vi "AlliGator Compute Phasor Plot Weber 2-Component Decomposition.vi"(5 "Lifetime Graph refnum":refnum<vi>, 8 "error in (no error)":errorcluster, 11 "AlliGator IV DVR":refnum<data-value>) -> (0 "error out":errorcluster, 1 "Message":string, 3 "AlliGator IV DVR":refnum<data-value>)   [LabVIEW 2021, in "AlliGator Phasor Plot.lvlib"]
doc: "Computes the 2-component linear decomposition of each phasor using Weber's apparoach.\n\nReturns two scatter plots (tau 2 vs tau 1 and f1 vs tau 1) sent to the Lifetime Graph."
uses:
  AlliGator Phasor Plot.lvlib
  Internal Variables/AlliGator Internal Variables v2.ctl
  <vilib>/vision/Image Controls.llb/IMAQ Image.ctl
  Internal Variables/AlliGator Gate Image Set.ctl
  Files/AlliGator FLI Dataset Type.ctl
  Files/AlliGator Data Series Type.ctl
  Dual-Channel Datasets/AlliGator Dataset Channel.ctl
  Settings/AlliGator Gate Arithmetic.ctl
  Source Image/AlliGator Displayed Image.ctl
  Image/Named ROI Description.ctl
  Phasor Graph/AlliGator Decay Metadata v3.ctl
  Decay Analysis/Decay Preprocessing/AlliGator Decay Background Subtraction Info.ctl
  Decay Analysis/Decay Preprocessing/AlliGator Baseline Subtraction Method.ctl
  Graphs/XY Graph/XY Graph Plot Shift Parameters.ctl
  Graphs/XY Graph/XY Graph Plot Shift Method.ctl
  Decay Analysis/Decay Preprocessing/AlliGator Decay Extrapolation Parameters.ctl
  Phasor/Calibration Phasor (m, phi).ctl
  Phasor/Phasor Reference Series.ctl
  Phasor/Phasor Calibration Map v2.ctl
  Phasor/Phasor (g, s).ctl
  Phasor Graph/AlliGator Raw Phasor Plot Data v4.ctl
  Phasor/Phasor Standard Deviation Options.ctl
  AlliGator Phasor Multi-Harmonic Data.ctl
  Phasor/Phasor Harmonic Data.ctl
  Decay Fit Parameter Map/AlliGator Decay Fit Options & Parameters v2.ctl
  Fits/IRF(X)PSED/Decay Fit Options v2.ctl
  Fits/Decay Convolution/Decay Model.ctl
  Fits/Residual Type.ctl
  Fits/IRF(X)PSED/Fit Weights Type.ctl
  Fits/Non-linear Fitting Method v2.ctl
  Fits/Fit Calculation Method.ctl
  Fits/Non-linear Fitting Algorithm.ctl
  Decay Analysis/Decay Fit/AlliGator Decay Fit Parameter Constraints 2.ctl
  Fits/IRF(X)PSED/Decay Fit Parameters In List.ctl
  Fits/IRF(X)PSED/MLE Baseline Offset Type.ctl
  Decay Analysis/Decay Preprocessing/AlliGator Decay Preprocessing Parameters.ctl
  Fits/IRF(X)PSED/Decay Fit Parameters & Derived Quantities List v2.ctl
  Decay Fit Parameter Map/AlliGator Parameter Maps Data.ctl
  Globals, Variables, Constants/AlliGator Variables List.ctl
  Variant/Variant to Data/Variant to [I32].vi
  Graphs/XY Graph/XY Graph Add-Ons.lvlib
  Phasor/Phasor.lvlib
  Error/Error.lvlib
  Globals, Variables, Constants/AlliGator Globals, Variables & Constants.lvlib
  Variant/Variant to Data/Variant to Data.lvlib
  Phasor Harmonic/AlliGator Phasor Harmonics.lvlib
  Image/Image.lvlib
  Decay Analysis/Decay Preprocessing/AlliGator Decay Preprocessing.lvlib
  Phasor Graph/AlliGator Phasor Graph.lvlib
  Files/AlliGator Files.lvlib
  Internal Variables/AlliGator Internal Variables.lvlib
  Source Image/AlliGator Source Image.lvlib
  Fits/Fits.lvlib
  Decay Analysis/Decay Fit/AlliGator Decay Fit.lvlib
  Decay Fit Parameter Map/AlliGator Decay Fit Parameter Map.lvlib
  Settings/AlliGator Settings.lvlib
  Dual-Channel Datasets/AlliGator Dual-Channel Datasets.lvlib
panel:
  # "see the AlliGator License on the block diagram (Ctrl+E or Window:Show Block Diagram)"
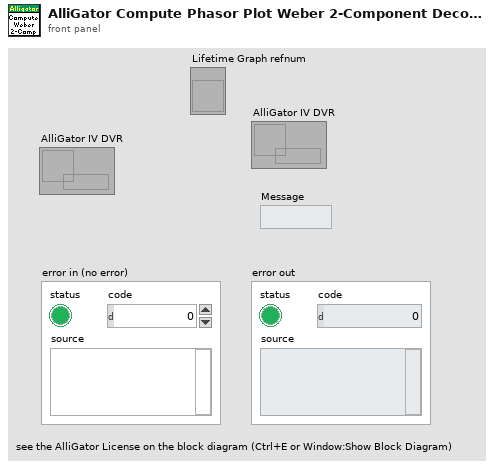
[diagram p1: front panel]
types:
  T1 = typedef "Phasor.lvlib/Phasor Harmonic Data.ctl" = cluster{"Phasor Harmonic Name":string, "Phasor Plot Settings Checksum":u64, "Phasor Frequency":dbl[unit], "Base Frequency":dbl[unit], "Harmonic Order":u8, "Phasor Plot Parameters":string, "Phasor Array [[CSG]]":csg[][], "Dataset File Path":path}
  T2 = typedef "AlliGator Globals, Variables & Constants.lvlib/AlliGator Variables List.ctl" = enum16{"---- GUI ----", "GUI:Initialization Status", "GUI:State Indicators Refnum", "GUI:Original AlliGator Menu Items", "GUI:Current Action Loop State", "GUI:Script in progress", "GUI:Playback", "GUI:Loop Playback", "GUI:Search ROI Used", "GUI:Search ROI", "Decay Graph Max Legend Size", "Intensity Graph Max Legend Size", "Decay Statistics Graph Max Legend Size", "Phasor Graph Max Legend Size", "Phasor Ratio Graph Max Legend Size", "Lifetime Graph Max Legend Size", "---- Files ----", "Files:Export Dataset Frames as Individual Files", "Files:Show Batch Export Help Balloons", "Files:Frames in Dataset", "Files:ptu File Frame Start Indices", "Files:Current Frame in Dataset", "Files:Current Frame Timestamp", "Files:Dataset Loaded", "Files:Dataset Metadata", "Files:Dataset Channel", "Files:Dataset Data Description", "Files:Background Dataset Metadata", "Files:Background Dataset Channel", "Files:Background Dataset Data Description", "Files:Background File Subtraction", "Files:Background File Path", "Files:Background File Pile-up Correction", "Files:Background File Pixel Well Capacity", "Files:Background File Scaling Factor", "Files:Current Dataset Load Settings", "Files:Dataset Path", "Files:ICCD-specific Information", "Files:Macrotime Gate Separation", "------ Python Plugins ------", "Python Plugins:Information", "Python Plugins:Python Session", "Python Plugins:Valid Python Session?", "---- Source Image ----", "Source Image:ROIs", "Source Image:Current ROI", "Source Image:ROI Event Refnum", "X_Source Image:Display Range", "X_Source Image:Palette Information", "X_Source Image:Type of Displayed Image", "X_Time Gate Slider", "Source Image:Palette List", "Source Image:Scale", "Source Image:ROI Overlay Color", "Source Image:Overlay to Erase", "Source Image:Is Displayed Image Accumulated", "Source Image:White Light Image Modified", "Source Image:Mask Image Modified", "---- Image Profile Window ----", "Image Profile:Window Event Refnum", "Image Profile:IntensityType", "Image Profile:Intensity Average Type", "Image Profile:Intensity-weighted SDV", "Image Profile:Box Profile Type", "Image Profile:Window Open", "Image Profile:Plotted Fit Parameter", "------ Phasor Graph -------", "Phasor Graph:Show Line", "---- Phasor Plot ---", "Phasor Plot:Parameters Changed", "Phasor Plot:FLI Dataset Modified since last Calculation", "Phasor Harmonics Data", "Selected Phasor Harmonics", "Phasor Harmonic Manager Event Refnum", "Phasor Plot:ROIs", "Phasor Plot:Current ROI", "Phasor Plot:ROI Event Refnum", "Phasor Plot:Image Reference Points", "Phasor Plot:Computed", "Phasor Plot:Palette Information", "Phasor Plot:Palette List", "Phasor Plot:Phasor Ratio Palette Information", "Phasor Plot:Phasor Ratio Palette List", "Phasor Plot:Image Scale", "Phasor Plot:Image Overlay to Erase", "Phasor Plot:Image Elements to Update", "Phasor Plot:Current Calculation Parameters", "Phasor Plot:Current Calibration Options", "Phasor Plot:Reset Cumulated Phasor Plot", "Phasor Plot:Reference 1", "Phasor Plot:Lifetime Reference 1", "Phasor Plot:Reference 1 Frequency", "Phasor Plot:Reference 2", "Phasor Plot:Lifetime Reference 2", "Phasor Plot:Reference 2 Frequency", "---- Decay Analysis ----", "Number of Selected Decays to Fit", "LS Fit Results", "LAR Fit Results", "BS Fit Results", "Last Decay Max - Min", "Best Fit Parameters", "Best Fit Parameter Names", "Actual Size X", "Actual Size Y", "Binning X", "Binning Y", "Actual # Gates", "Dataset Number", "Gates to...", "Gates Skipped", "Gates to keep", "Gate Step", "Gate Separation", "Reversed Gates", "Pile-up Correction", "Pixel Well Capacity", "Background Subtracted", "Background Subtraction Method", "Background Definition Range", "Background File (deprecated)", "Number of Dataset Accumulated", "Array of Accumulated Dataset Paths", "Do Averaged Datasets", "Destination File Path", "Process Plot Target", "Use 1/D as Phasor Frequency", "---- Decay Fit Parameter Map -----", "Decay Fit Parameter Map:Palette Information", "Decay Fit Parameter Map:Palette List", "Decay Fit Parameter Map:X Resolution", "Decay Fit Parameter Map:Y Resolution", "---- Parameter Map ----", "Parameter Map:Palette Information", "Parameter Map:Palette List", "------- Local Decay Window ---------", "Local Decay Graph Window:Event Refnum", "Local Decay Graph Window:Use normalized IRF for convolution", "----- Miscellaneous ----", "Misc:Skippable Dialog Windows Status"}
  T3 = typedef "AlliGator Internal Variables.lvlib/AlliGator Internal Variables v2.ctl" = cluster{"Displayed Image":T4, "White Light Image":T4, "Mask Image":T4, "ROI Mask Image":T4, "Current Dataset Images 1":T5, "Background Dataset Images 1":T5, "Current Dataset Images 2":T5, "Background Dataset Images 2":T5, "Current Dataset Arithmetic Images":T5, "Accumulated Dataset Images 1":T5, "Accumulated Dataset Images 2":T5, "Accumulated Dataset Arithmetic Images":T5, "Phasor Plot Image":T4, "Decay Fit Parameter Map Image":T4, "Parameter Map Image":T4, "Single Data Point Path":path, "White Light Image Path":path, "Mask Image Path":path, "Time-Series Folder":path, "[Time-Series Paths]":path[], "Current Dataset":i32, "Single Dataset Type":T6, "Current Folder":string, "AlliGator Data Series Type":T7, "# Datasets":i32, "Dual-Channel Dataset":bool, "Selected Channel Name":string, "Dataset Channel":T8, "Channel Arithmetic":T9, "Dual-Channel Background Dataset":bool, "Background Channel":T8, "Dual-Channel Accumulated Dataset":bool, "Start Time":dbl, "[Time-Series Timestamps]":dbl[], "[Intensity Corrections]":dbl[], "Time Series Script":bool, "Type of Displayed Image":T10, "Gate Image Slide":u16, "# Gates":i32, "ROIs":T11[], "ROI Decay":cluster{"t Array":dbl[], "I Array":dbl[]}, "Valid Decay":bool, "Decay  Metadata":T13, "Reference Decay Plot Name":string, "Reference Decay":cluster{"t Array":dbl[], "I Array":dbl[]}, "Decay Shift Plot":cluster{"Time Stamps":dbl[], "Decay Shifts":dbl[]}, "[Decays Max Values]":sgl[], "[Decays Min Values]":sgl[], "Calibration Phasor":T19, "Calibration Phasor Series":T20, "Phasor Calibration Map":T21, "Calibration Map MD5 Digest":string, "Last Raw Phasor":T22, "Last Calibrated Phasor":T22, "Last Calibrated Phasor SDV":T22, "Phasor Graph:Phasor Plot":cluster{"g Array":dbl[], "s Array":dbl[]}, "Phasor Graph:Phasor SDV Plot":cluster{"g Array":dbl[], "s Array":dbl[]}, "[Phasor Graph:Raw Phasor Plots]":T23[], "Phasor Plot locked to Ref 1":i32, "[Phasor Plot(s) locked to Ref 1]":i32[], "[Phasor Plot(s) locked to Ref 2]":i32[], "[Pixel Phasors]":T22[], "[[Sum Image]]":dbl[][], "[[CSG Phasors]]":csg[][], "[[Valid Pixel?]]":bool[][], "I/m/phi Dataset":cluster{"I/m/phi Dataset?":bool, "Base Frequency":dbl[unit], "Harmonic Orders":u8[]}, "Multi Phasor Plot Data":T25, "Decay Fit Options & Parameters":T26, "Fit Options: Decay Preprocessing Parameters":T37, "Fit Options: Reference Decay":cluster{"t Array":dbl[], "I Array":dbl[]}, "Is Full Image Parameters Map":bool, "Is Single-Pixels Parameters Map":bool, "NLSF Parameters Map X Resolution":i32, "NLSF Parameters Map Y Resolution":i32, "[Single Decay Fit Parameters]":dbl[], "Fit Model":T28, "[[Multiple Decays Fit Parameters]]":dbl[][], "[[Multiple Decays Fit Parameter SDVs]]":dbl[][], "[[IRFs]]":dbl[][], "IRF Array Time Axis":dbl[], "Decay Array Time Axis":dbl[], "[Decay Fit Parameter Names]":T38[], "[[Phasor Ratios]]":dbl[][], "[[Average Lifetimes]]":dbl[][], "Amplitude Weighted Average Lifetime":bool, "[Decay Sum]":dbl[], "[Map Set Names]":string[], "[Parameter Maps]":T39[], "[[User-defined Quantities]]":dbl[][], "User-defined Quantity":string}
  T4 = typedef "IMAQ Image.ctl" = refnum<image>
  T5 = typedef "AlliGator Internal Variables.lvlib/AlliGator Gate Image Set.ctl" = cluster{"SGL Image Max":T4, "SGL Image Sum":T4, "SGL Gate Images":T4[], "SGL Image Min":T4}
  T6 = typedef "AlliGator Files.lvlib/AlliGator FLI Dataset Type.ctl" = enum16{"HDF5 FLI Dataset", "Gate Image Folder", ".sdt FLI Dataset (Becker & Hickl)", ".ptu FLI Dataset (PicoQuant)", "SS1 FLI Dataset", "SS2 FLI Dataset", "I/m/phi Dataset", ".bin FLI Dataset (PicoQuant Binned)", ".bin FLI Dataset (Piccolo Binned)", ".mat FLI Dataset"}
  T7 = typedef "AlliGator Files.lvlib/AlliGator Data Series Type.ctl" = enum16{"Not a Supported Series", "Gate Images Folder Series", "SwissSPAD 2 Dataset Series", "B&H FLI Dataset Series", "PicoQuant PTU FLI Dataset Series", "PicoQuant BIN FLI Dataset Series", "Piccolo hist BIN FLI Dataset Series", "HDF5 FLI Dataset Series"}
  T8 = typedef "AlliGator Dual-Channel Datasets.lvlib/AlliGator Dataset Channel.ctl" = enum16{"G2", "INT"}
  T9 = typedef "AlliGator Settings.lvlib/AlliGator Gate Arithmetic.ctl" = enum16{"None", "INT-G2", "G2/INT*<INT>", "(1 - G2/INT)*<INT>"}
  T10 = typedef "AlliGator Source Image.lvlib/AlliGator Displayed Image.ctl" = enum16{"Single Gate", "Sum of All Gates", "Max of All Gates", "Min of All Gates", "-", "White Ligth Image", "Mask Image"}
  T11 = typedef "Image.lvlib/Named ROI Description.ctl" = cluster{"ROI Descriptor":T12, "ROI Name":string, "Overlay Color":u32}
  T12 = typedef "ROI Descriptor" = cluster{"Global Rectangle":i32[], "Contours":cluster{"ID":enum32{"External", "Internal"}, "Type":u32, "Coordinates":i32[]}[]}
  T13 = typedef "AlliGator Phasor Graph.lvlib/AlliGator Decay Metadata v3.ctl" = cluster{"ROI Descriptor":T12, "ROI Center":cluster{"X":i32, "Y":i32}, "Decay Background Subtraction Info":T14, "Decay Reverted":bool, "Decay Smoothened":bool, "Decay Straightened":bool, "Fitted Tau (Decay Straightening)":dbl, "Decay Shift Parameters":T16, "Decay Shifted":bool, "Decay Extrapolated":bool, "Decay Extrapolation Parameters":T18, "Decay Normalized":bool, "Fold Decay":bool, "# Folds":u32}
  T14 = typedef "AlliGator Decay Preprocessing.lvlib/AlliGator Decay Background Subtraction Info.ctl" = cluster{"Laser Period":dbl[unit], "Gate Duration":dbl[unit], "Baseline Subtraction Method":T15, "Background Definition Range":cluster{"Min Gate":dbl[unit], "Max Gate":dbl[unit]}, "Total Intensity w/o Bkgd Subtraction":dbl, "Bkgd-subtracted Intensity (exp)":dbl, "# Data Points":i32, "Background/Gate":dbl, "Fitted Lifetime":dbl[unit], "Bkgd-subtracted Intensity (theo)":dbl}
  T15 = typedef "AlliGator Decay Preprocessing.lvlib/AlliGator Baseline Subtraction Method.ctl" = enum16{"Mean", "Min", "Square Gated Single-Exponential", "File", "Constant"}
  T16 = typedef "XY Graph Add-Ons.lvlib/XY Graph Plot Shift Parameters.ctl" = cluster{"Type":T17, "Shift":dbl[unit], "Threshold":dbl, "Rotate":bool}
  T17 = typedef "XY Graph Add-Ons.lvlib/XY Graph Plot Shift Method.ctl" = enum16{"Default", "CFD", "Threshold", "Cross-Correlation"}
  T18 = typedef "AlliGator Decay Preprocessing.lvlib/AlliGator Decay Extrapolation Parameters.ctl" = cluster{"Additional Points":u32, "Head Fraction":dbl, "Fitted Tau":dbl, "Use Periodicity":bool, "Use Cursors":bool, "Tail Fraction":dbl}
  T19 = typedef "Phasor.lvlib/Calibration Phasor (m, phi).ctl" = cluster{"m":dbl, "phi":dbl, "Phasor Frequency":dbl[unit], "Reference Lifetime":dbl[unit]}
  T20 = typedef "Phasor.lvlib/Phasor Reference Series.ctl" = cluster{"m Array":dbl[], "phi Array":dbl[], "Phasor Frequency":dbl[unit], "Calibration Lifetime":dbl[unit]}
  T21 = typedef "Phasor.lvlib/Phasor Calibration Map v2.ctl" = cluster{"Phasor Frequency":dbl[unit], "Calibration Lifetime":dbl[unit], "ROI Centers":cluster{"X":i32, "Y":i32}[], "ROI Descriptors":T12[], "Map Resolution X":i32, "Map Resolution Y":i32, "z Array":cdb[]}
  T22 = typedef "Phasor.lvlib/Phasor (g, s).ctl" = cluster{"g":dbl, "s":dbl}
  T23 = typedef "AlliGator Phasor Graph.lvlib/AlliGator Raw Phasor Plot Data v4.ctl" = cluster{"Phasor Plot Name":string, "Raw Phasor Plot":T22[], "Phasor Frequency":dbl[unit], "[Decay Metadata]":T13[], "Raw Phasor Plot SDV":T22[], "Phasor SDV Options":T24, "[Calibration Phasor]":T19[]}
  T24 = typedef "Phasor.lvlib/Phasor Standard Deviation Options.ctl" = cluster{"Compute Estimated SDV":bool, "# Replicas":u32, "Use Estimated Average Phasor":bool}
  T25 = typedef "AlliGator Phasor Plot.lvlib/AlliGator Phasor Multi-Harmonic Data.ctl" = cluster{"Base Frequency":dbl[unit], "# Harmonics":u8, "Harmonic Orders":u8[], "Phasor Plot Settings Checksum":u64, "Phasor Harmonic Data Array":T1[]}
  T26 = typedef "AlliGator Decay Fit Parameter Map.lvlib/AlliGator Decay Fit Options & Parameters v2.ctl" = cluster{"SYNC Period":dbl[unit], "Fit Options":T27, "Fit Parameter Constraints":T34[], "MLE Baseline Offset":dbl, "MLE Baseline Offset Type":T36}
  T27 = typedef "Fits.lvlib/Decay Fit Options v2.ctl" = cluster{"Show Fit Residuals":bool, "Fit Model":T28, "Residual Type":T29, "Max Decay Percentile":dbl, "Min Decay Percentile":dbl, "Show Full Decay":bool, "Weights":T30, "Fitting Method":T31, "Compute Parameter Uncertainties":bool, "Periodic Boundaries":bool, "Model Calculation":T32, "Period":dbl[unit], "Termination Criteria":cluster{"Max Iterations":i32, "Max Function Calls":i32, "Max Time":dbl[unit], "Function Tolerance":dbl, "Parameter Tolerance":dbl, "Gradient Tolerance":dbl, "Min Lambda":dbl, "Max Lambda":dbl, "Initial Tick Count":u32}, "Offset Resolution":dbl[unit], "Use Local IRF":bool, "Fitting Algorithm":T33}
  T28 = typedef "Fits.lvlib/Decay Model.ctl" = enum16{"1-Exponential", "2-Exponentials"}
  T29 = typedef "Fits.lvlib/Residual Type.ctl" = enum16{"Standard", "Normalized", "Reduced"}
  T30 = typedef "Fits.lvlib/Fit Weights Type.ctl" = enum16{"Unweighted", "1/Variance", "Best of All"}
  T31 = typedef "Fits.lvlib/Non-linear Fitting Method v2.ctl" = enum16{"Least Square", "Least Absolute Residual", "Bisquare", "MLE", "-", "Best of All"}
  T32 = typedef "Fits.lvlib/Fit Calculation Method.ctl" = enum16{"Simulation", "Convolution", "Integration"}
  T33 = typedef "Fits.lvlib/Non-linear Fitting Algorithm.ctl" = enum16{"Levenberg-Marquardt", "Trust-Region Dogleg"}
  T34 = typedef "AlliGator Decay Fit.lvlib/AlliGator Decay Fit Parameter Constraints 2.ctl" = cluster{"Fit Parameter":T35, "Min Value":dbl, "Max Value":dbl, "Global":bool, "Used":bool}
  T35 = typedef "Fits.lvlib/Decay Fit Parameters In List.ctl" = enum16{"Offset", "Baseline", "A_1", "tau_1", "A_2", "tau_2"}
  T36 = typedef "Fits.lvlib/MLE Baseline Offset Type.ctl" = enum32{"Absolute", "Percentage"}
  T37 = typedef "AlliGator Decay Preprocessing.lvlib/AlliGator Decay Preprocessing Parameters.ctl" = cluster{"Background Subtraction":bool, "Straighten Decay":bool, "Reverse Gates":bool, "1-Normalized Decay":bool, "Smoothen Decay":bool, "Smoothing Parameter":dbl, "Shift Decay":bool, "Decay Shift Parameters":T16, "Extrapolate Decay":bool, "Additional Points":u32, "Head Fraction":dbl, "Pixel-Normalize Decay":bool, "Use Periodicity":bool, "Use Cursors":bool, "Tail Fraction":dbl, "Use Decay Pre-Processing":bool, "Fold Decay":bool, "# Folds":u32, "[0-1]-Normalized Decay":bool}
  T38 = typedef "Fits.lvlib/Decay Fit Parameters & Derived Quantities List v2.ctl" = enum16{"Offset", "Baseline", "A_1", "tau_1", "A_2", "tau_2", "<tau>_a", "f1_a", "f2_a", "<tau>_i", "f1_i", "f2_i", "-", "R^2", "Chi^2"}
  T39 = typedef "AlliGator Decay Fit Parameter Map.lvlib/AlliGator Parameter Maps Data.ctl" = cluster{"Map Set Name":string, "[Parameter Names]":string[], "[[Parameters]]":dbl[][], "[[Parameter SDVs]]":dbl[][], "Decay Array Time Axis":dbl[], "[[IRFs]]":dbl[][], "IRF Array Time Axis":dbl[]}
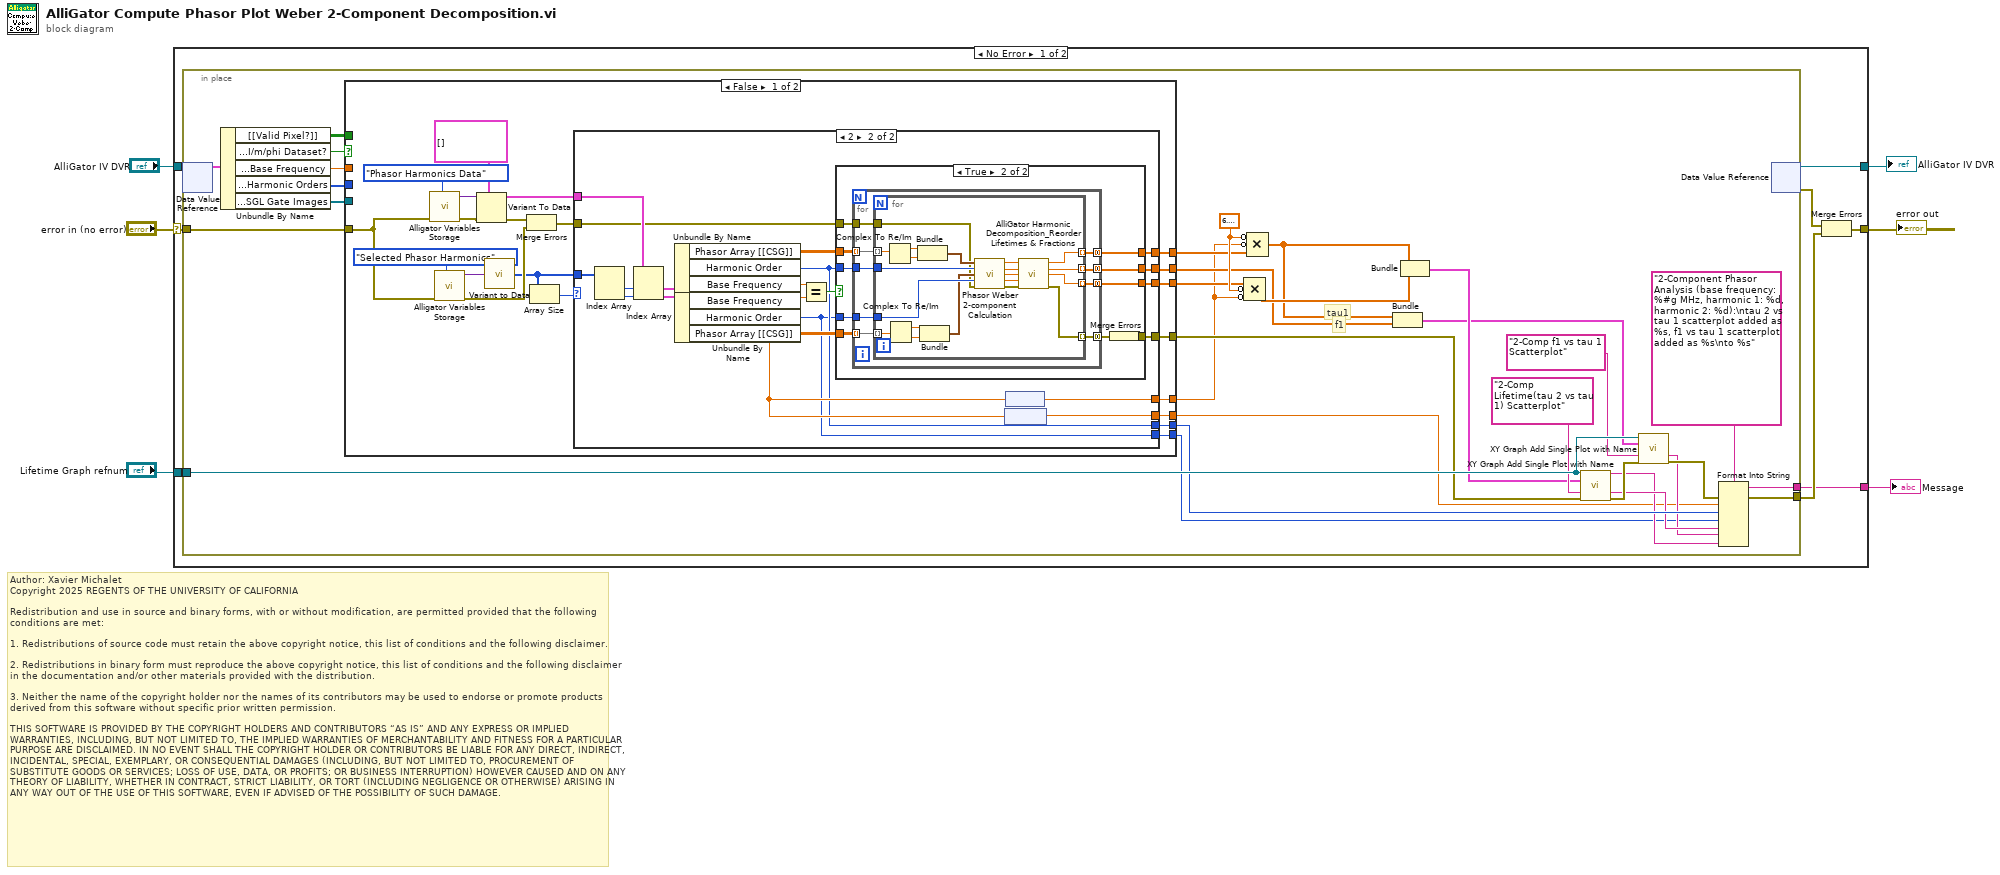
[diagram p0: block diagram]
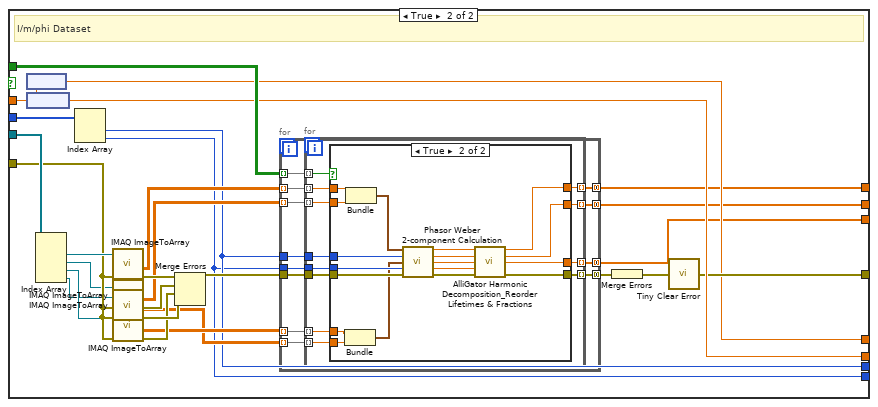
[diagram p4: hidden frame]
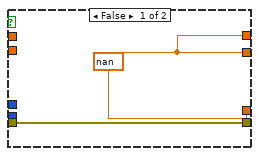
[diagram p5: hidden frame]
diagram:
  # "Author: Xavier Michalet\nCopyright 2025 REGENTS OF THE UNIVERSITY OF CALIFORNIA\n\nRedistribution and use in source and binary forms, with or without modification, are permitted provided that the following conditions are met:\n\n1. Redistributions of source code must retain the above copyright notice, this list of conditions and the following disclaimer.\n\n2. Redistributions in binary form must reproduce the above copyright notice, this list of conditions and the following disclaimer in the documentation and/or other materials provided with the distribution.\n\n3. Neither the name of the copyright holder nor the names of its contributors may be used to endorse or promote products derived from this software without specific prior written permission.\n\nTHIS SOFTWARE IS PROVIDED BY THE COPYRIGHT HOLDERS AND CONTRIBUTORS “AS IS” AND ANY EXPRESS OR IMPLIED WARRANTIES, INCLUDING, BUT NOT LIMITED TO, THE IMPLIED WARRANTIES OF MERCHANTABILITY AND FITNESS FOR A PARTICULAR PURPOSE ARE DISCLAIMED. IN NO EVENT SHALL THE COPYRIGHT HOLDER OR CONTRIBUTORS BE LIABLE FOR ANY DIRECT, INDIRECT, INCIDENTAL, SPECIAL, EXEMPLARY, OR CONSEQUENTIAL DAMAGES (INCLUDING, BUT NOT LIMITED TO, PROCUREMENT OF SUBSTITUTE GOODS OR SERVICES; LOSS OF USE, DATA, OR PROFITS; OR BUSINESS INTERRUPTION) HOWEVER CAUSED AND ON ANY THEORY OF LIABILITY, WHETHER IN CONTRACT, STRICT LIABILITY, OR TORT (INCLUDING NEGLIGENCE OR OTHERWISE) ARISING IN ANY WAY OUT OF THE USE OF THIS SOFTWARE, EVEN IF ADVISED OF THE POSSIBILITY OF SUCH DAMAGE."
  n1 = case shown="No Error" "error in (no error)" {
    selector: "error in (no error)" -> [w10 w198]
    tunnel: "AlliGator IV DVR" -> [w14 w199]
    tunnel: [w13 w199] -> w5
    tunnel: [w9 w198] -> w1
    tunnel: "Lifetime Graph refnum" -> [w11 _]
    tunnel: [w7 _] -> w2
    frame No Error {
      n2 = in-place {
        in-place-border: w11 -> [w44]
        in-place-border: w10 -> [w43]
        in-place-border: [w42] -> w8
        in-place-border: [w41] -> w7
        w24 = 6.283185307179586
        # "f1"
        # "tau1"
        n3 = in-place-dvr #1(w14) -> (w45:T3)  [unwired: 1 out]
        n4 = Unbundle By Name(w45) -> ("[[Valid Pixel?]]"=w38:bool[][], "I/m/phi Dataset.I/m/phi Dataset?"=w25:bool, "I/m/phi Dataset.Base Frequency"=w37:dbl[unit], "I/m/phi Dataset.Harmonic Orders"=w39:u8[], "Current Dataset Images 1.SGL Gate Images"=w40:T4[])
        n5 = case shown="False" w25 {
          tunnel: w40 -> [_ w153]
          tunnel: w39 -> [_ w152]
          tunnel: w38 -> [_ w151]
          tunnel: w43 -> [w61 w149]
          tunnel: w37 -> [_ w135]
          tunnel: [w48 w134] -> w16
          tunnel: [w47 w133] -> w31
          tunnel: [w50 w132] -> w27
          tunnel: [w46 w130] -> w26
          tunnel: [w53 w128] -> w21
          tunnel: [w52 w127] -> w20
          tunnel: [w51 w126] -> w19
          tunnel: [w49 w129] -> w15
          frame False {
            n6 = call "Alligator Variables Storage.vi"("AlliGator Variable"=AlliGator_Variables_List."Phasor Harmonics Data" ("Alligator Variable"), "Error In"=w61) -> ("Error Out"=w63:errorcluster, "Data out"=w62:variant)  [unwired: 7 in, 1 out]
            n7 = call "Alligator Variables Storage.vi"("AlliGator Variable"=AlliGator_Variables_List."Selected Phasor Harmonics" ("Alligator Variable"), "Error In"=w61) -> ("Error Out"=w56:errorcluster, "Data out"=w64:variant)  [unwired: 7 in, 1 out]
            n8 = Variant To Data(error in=w63, type=T1[] [] ("Array"), Variant=w62) -> (data=w58:T1[], error out=w57:errorcluster)
            n9 = call-poly "Variant to Data.vi"("Variant"=w64) -> ("Value"=w54:i32[])  [unwired: 8 in]
            n10 = Merge Errors(w57, w56) -> (w55:errorcluster)
            n11 = Array Size(array=w54) -> (size(s)=w59:i32)
            n12 = case shown="2" w59 {
              tunnel: w58 -> [_ w85]
              tunnel: w55 -> [_ w72]
              tunnel: w54 -> [_ w86]
              tunnel: [_ w76] -> w53
              tunnel: [_ w75] -> w52
              tunnel: [_ w74] -> w51
              tunnel: [_ w73] -> w50
              tunnel: [_ w71] -> w49
              tunnel: [_ w69] -> w48
              tunnel: [_ w68] -> w47
              tunnel: [_ w67] -> w46
              frame 0, Default {
              }
              frame 2 {
                n13 = Index Array(array=w86) -> (element #1=w84:i32, element #2=w83:i32)  [unwired: 2 in]
                n14 = Index Array(array=w85, index #1=w84, index #2=w83) -> (element #1=w82:T1, element #2=w81:T1)
                n15 = Unbundle By Name(w82) -> ("Phasor Array [[CSG]]"=w77:csg[][], "Harmonic Order"=w68:u8, "Base Frequency"=w80:dbl[unit])
                n16 = Unbundle By Name(w81) -> ("Base Frequency"=w70:dbl[unit], "Harmonic Order"=w67:u8, "Phasor Array [[CSG]]"=w78:csg[][])
                n17 = Equal?(x=w80, y=w70) -> (x = y?=w79:bool)
                n18 = case shown="True" w79 {
                  tunnel: w68 -> [_ w96]
                  tunnel: w67 -> [_ w95]
                  tunnel: w78 -> [_ w93]
                  tunnel: w77 -> [_ w94]
                  tunnel: [_ w92] -> w76
                  tunnel: [_ w91] -> w75
                  tunnel: [_ w90] -> w74
                  tunnel: [_ w88] -> w73
                  tunnel: w72 -> [_ w87]
                  frame False {
                  }
                  frame True {
                    n19 = for {
                      tunnel: w96 -> [w105]
                      tunnel: w95 -> [w104]
                      tunnel: w94 -> [w103] mode=indexing
                      tunnel: w93 -> [w102] mode=indexing
                      tunnel: [w101] -> w92 mode=concatenating
                      tunnel: [w100] -> w91 mode=concatenating
                      tunnel: [w99] -> w90 mode=concatenating
                      tunnel: [w98] -> w89 mode=concatenating
                      tunnel: w87 -> [w97]
                      n20 = for {
                        tunnel: w105 -> [w121]
                        tunnel: w104 -> [w120]
                        tunnel: w103 -> [w119] mode=indexing
                        tunnel: w102 -> [w118] mode=indexing
                        tunnel: [w111] -> w101 mode=indexing
                        tunnel: [w110] -> w100 mode=indexing
                        tunnel: [w109] -> w99 mode=indexing
                        tunnel: [w107] -> w98 mode=indexing
                        tunnel: w97 -> [w106]
                        n21 = Complex To Re/Im(x + iy=w119) -> (x=w117:sgl, y=w116:sgl)
                        n22 = Complex To Re/Im(x + iy=w118) -> (x=w114:sgl, y=w113:sgl)
                        n23 = Bundle(w117, w116) -> (w115:cluster{sgl, sgl})  [unwired: 1 in]
                        n24 = Bundle(w114, w113) -> (w112:cluster{sgl, sgl})  [unwired: 1 in]
                        n25 = call "Phasor Weber 2-component Calculation.vi"("Phasor 1 (g, s)"=w115, "Harmonic Order 1"=w121, "Phasor 2 (g, s)"=w112, "Harmonic Order 2"=w120, "Error In"=w106) -> ("Reduced Lifetime 1"=w125:dbl, "Fraction 1"=w123:dbl, "Reduced Lifetime 2"=w124:dbl, "Fraction 2"=w122:dbl, "Error Out"=w108:errorcluster)  [unwired: 6 in]
                        n26 = call "AlliGator Harmonic Decomposition_Reorder Lifetimes & Fractions.vi"("Reduced Lifetime 1"=w125, "Fraction 1"=w123, "Reduced Lifetime 2"=w124, "Fraction 2"=w122, "Error In"=w108) -> ("Smallest Reduced Lifetime (1)"=w111:dbl, "Fraction 1"=w110:dbl, "Largest Reduced Lifetime (2)"=w109:dbl, "Error Out"=w107:errorcluster)  [unwired: 6 in, 1 out]
                      }
                    }
                    n27 = Merge Errors(w89) -> (w88:errorcluster)
                  }
                }
                n28 = node(w70) -> (w69:dbl)
                n29 = node(w70) -> (w71:dbl)
              }
            }
          }
          frame True {
            # "I/m/phi Dataset"
            n30 = node(w135) -> (w129:dbl)
            n31 = node(w135) -> (w134:dbl)
            n32 = Index Array(array=w153) -> (element #1=w150:T4, element #2=w148:T4, element #3=w147:T4, element #4=w146:T4)  [unwired: 4 in]
            n33 = Index Array(array=w152) -> (element #1=w133:u8, element #2=w130:u8)  [unwired: 2 in]
            n34 = call "IMAQ ImageToArray"("error in (no error)"=w149, "Image"=w150) -> ("Image Pixels (Float)"=w140:sgl[][], "error out"=w145:errorcluster)  [unwired: 2 in, 3 out]
            n35 = call "IMAQ ImageToArray"("error in (no error)"=w149, "Image"=w148) -> ("Image Pixels (Float)"=w139:sgl[][], "error out"=w142:errorcluster)  [unwired: 2 in, 3 out]
            n36 = call "IMAQ ImageToArray"("error in (no error)"=w149, "Image"=w146) -> ("Image Pixels (Float)"=w137:sgl[][], "error out"=w144:errorcluster)  [unwired: 2 in, 3 out]
            n37 = call "IMAQ ImageToArray"("error in (no error)"=w149, "Image"=w147) -> ("Image Pixels (Float)"=w138:sgl[][], "error out"=w143:errorcluster)  [unwired: 2 in, 3 out]
            n38 = Merge Errors(w145, w142, w143, w144) -> (w141:errorcluster)
            n39 = for {
              tunnel: w133 -> [w165]
              tunnel: w130 -> [w164]
              tunnel: w151 -> [w163] mode=indexing
              tunnel: [w162] -> w128 mode=concatenating
              tunnel: [w161] -> w126 mode=concatenating
              tunnel: [w160] -> w127 mode=concatenating
              tunnel: w141 -> [w159]
              tunnel: w140 -> [w158] mode=indexing
              tunnel: w139 -> [w157] mode=indexing
              tunnel: w138 -> [w156] mode=indexing
              tunnel: w137 -> [w155] mode=indexing
              tunnel: [w154] -> w136 mode=concatenating
              n40 = for {
                tunnel: w165 -> [w177]
                tunnel: w164 -> [w176]
                tunnel: w163 -> [w166] mode=indexing
                tunnel: [w175] -> w162 mode=indexing
                tunnel: [w174] -> w161 mode=indexing
                tunnel: [w173] -> w160 mode=indexing
                tunnel: w159 -> [w172]
                tunnel: w158 -> [w171] mode=indexing
                tunnel: w157 -> [w170] mode=indexing
                tunnel: w156 -> [w169] mode=indexing
                tunnel: w155 -> [w168] mode=indexing
                tunnel: [w167] -> w154 mode=indexing
                n41 = case shown="True" w166 {
                  tunnel: w177 -> [_ w197]
                  tunnel: w176 -> [_ w196]
                  tunnel: [w178 w188] -> w175
                  tunnel: [w178 w186] -> w174
                  tunnel: [w178 w183] -> w173
                  tunnel: w172 -> [w179 w195]
                  tunnel: w171 -> [_ w194]
                  tunnel: w170 -> [_ w193]
                  tunnel: w169 -> [_ w191]
                  tunnel: w168 -> [_ w190]
                  tunnel: [w179 w180] -> w167
                  frame False {
                    w178 = nan ("Reduced Lifetime 1")
                  }
                  frame True {
                    n42 = Bundle(w191, w190) -> (w189:cluster{sgl, sgl})  [unwired: 1 in]
                    n43 = Bundle(w194, w193) -> (w192:cluster{sgl, sgl})  [unwired: 1 in]
                    n44 = call "Phasor Weber 2-component Calculation.vi"("Phasor 1 (g, s)"=w192, "Harmonic Order 1"=w197, "Phasor 2 (g, s)"=w189, "Harmonic Order 2"=w196, "Error In"=w195) -> ("Reduced Lifetime 1"=w187:dbl, "Fraction 1"=w184:dbl, "Reduced Lifetime 2"=w185:dbl, "Fraction 2"=w182:dbl, "Error Out"=w181:errorcluster)  [unwired: 6 in]
                    n45 = call "AlliGator Harmonic Decomposition_Reorder Lifetimes & Fractions.vi"("Reduced Lifetime 1"=w187, "Fraction 1"=w184, "Reduced Lifetime 2"=w185, "Fraction 2"=w182, "Error In"=w181) -> ("Smallest Reduced Lifetime (1)"=w188:dbl, "Fraction 1"=w183:dbl, "Largest Reduced Lifetime (2)"=w186:dbl, "Error Out"=w180:errorcluster)  [unwired: 6 in, 1 out]
                  }
                }
              }
            }
            n46 = Merge Errors(w136) -> (w131:errorcluster)
            n47 = call "Tiny Clear Error.vi"("Error In"=w131) -> ("no Error Out"=w132:errorcluster)  [unwired: 8 in]
          }
        }
        n48 = Compound Arithmetic op=MULTIPLY(w19, invert w24, invert w15) -> (w23:dbl[])
        n49 = Compound Arithmetic op=MULTIPLY(invert w24, invert w15, w21) -> (w22:dbl[])
        n50 = Bundle(w22, w20) -> (w17:cluster{dbl[], dbl[]})  [unwired: 1 in]
        n51 = Bundle(w22, w23) -> (w18:cluster{dbl[], dbl[]})  [unwired: 1 in]
        n52 = call "XY Graph Add Single Plot with Name.vi"("XYGraph Ref in"=w44, "Plot"=w18, "Plot Name (\"Plot\")"="2-Comp Lifetime(tau 2 vs tau 1) Scatterplot" ("New Name"), "error in (no error)"=w27) -> ("XY Graph Caption (or Label)"=w28:string, "Plot Name"=w30:string, "error out"=w34:errorcluster)  [unwired: 8 in, 1 out]
        n53 = call "XY Graph Add Single Plot with Name.vi"("XYGraph Ref in"=w44, "Plot"=w17, "Plot Name (\"Plot\")"="2-Comp f1 vs tau 1 Scatterplot" ("New Name"), "error in (no error)"=w34) -> ("Plot Name"=w29:string, "error out"=w32:errorcluster)  [unwired: 8 in, 2 out]
        n54 = Format Into String(format string="2-Component Phasor Analysis (base frequency: %#g MHz, harmonic 1: %d, harmonic 2: %d):\ntau 2 vs tau 1 scatterplot added as %s, f1 vs tau 1 scatterplot added as %s\nto %s", error in=w32, w16, w31, w26, w30, w29, w28) -> (resulting string=w41:string, error out=w42:errorcluster)  [unwired: 1 in]
        n55 = in-place-dvr #1() -> (w13:refnum<data-value>, w12:errorcluster)  [unwired: 1 in]
      }
      n56 = Merge Errors(w12, w8) -> (w9:errorcluster)
    }
    frame Error {
    }
  }
  "error out" <- w1
  "AlliGator IV DVR" <- w5
  "Message" <- w2
